vi "Delete Operations.vi"(8 "error in (no error)":errorcluster caption="entrée d'erreur (pas d'erreur)", 10 "key":variant, 11 "Operations en entrée":refnum<class "Operations.lvclass"> caption="DNL_LabVIEW Object in") -> (0 "error out":errorcluster caption="sortie d'erreur", 3 "Operations en sortie":refnum<class "Operations.lvclass"> caption="DNL_LabVIEW Object out")   [LabVIEW 2012, in "Operations.lvclass"]
uses:
  Operations.lvclass
  Operations.lvclass/Operations.ctl
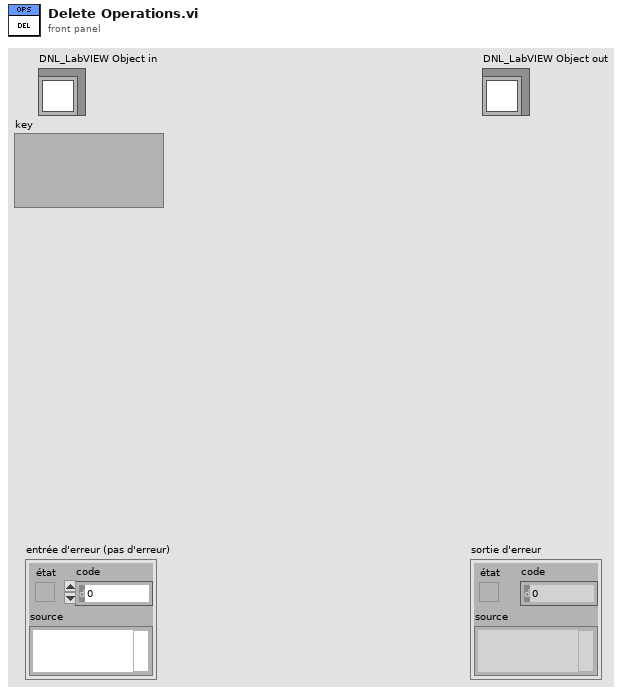
[diagram p1: front panel]
types:
  T1 = typedef "Dictionary Object RefNum__ogtk.ctl" = refnum<k1>
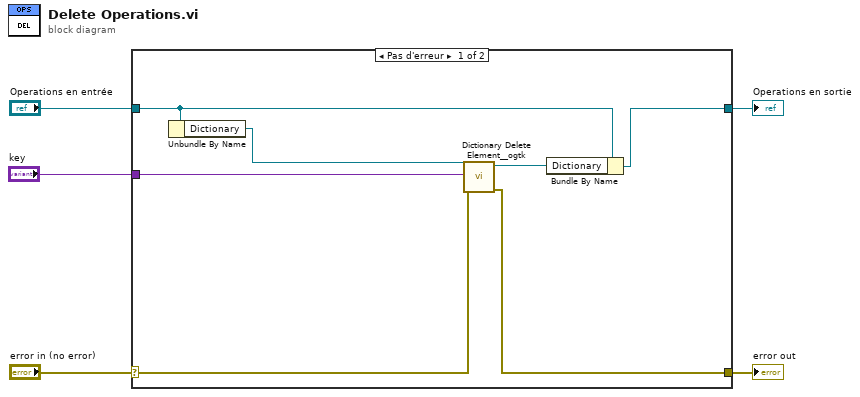
[diagram p0: block diagram]
diagram:
  n1 = case shown="Pas d'erreur" "error in (no error)" {
    selector: "error in (no error)" -> [w7 w14]
    tunnel: [w9 w14] -> w4
    tunnel: [w11 w13] -> w2
    tunnel: "Operations en entrée" -> [w12 w13]
    tunnel: "key" -> [w6 _]
    frame No Error {
      n2 = Unbundle By Name(w12) -> ("Dictionary"=w8:T1)
      n3 = call <userlib>:"Dictionary Delete Element__ogtk.vi"("error in (no error)"=w7, "key"=w6, "dictionary"=w8) -> ("error out"=w9:errorcluster, "dictionary out"=w10:T1)  [unwired: 7 in]
      n4 = Bundle By Name(cluster=w12, "Dictionary"=w10) -> (w11:refnum<class "Operations.lvclass">)
    }
    frame Error {
    }
  }
  "error out" <- w4
  "Operations en sortie" <- w2
